vi "HW#1.vi"() -> ()   [LabVIEW 2018]
panel:
  out "Time":timestamp
  out "XY Graph":cluster{"X":dbl, "Y":dbl}[](graph)
  in  "File":path
  in  "Clear":bool
  in  "Plot Data":bool
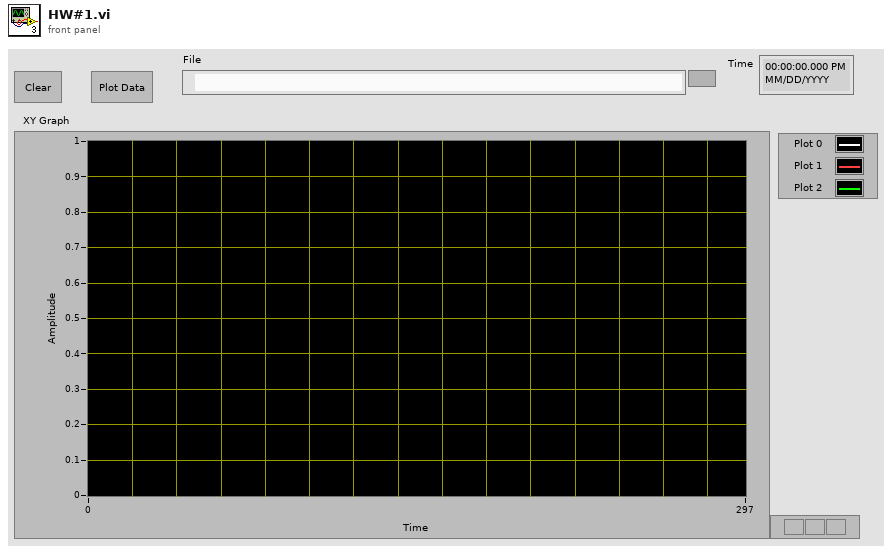
[diagram p1: front panel]
types:
  T1 = cluster{"Duration":u32, "State":bool, "Running":bool}
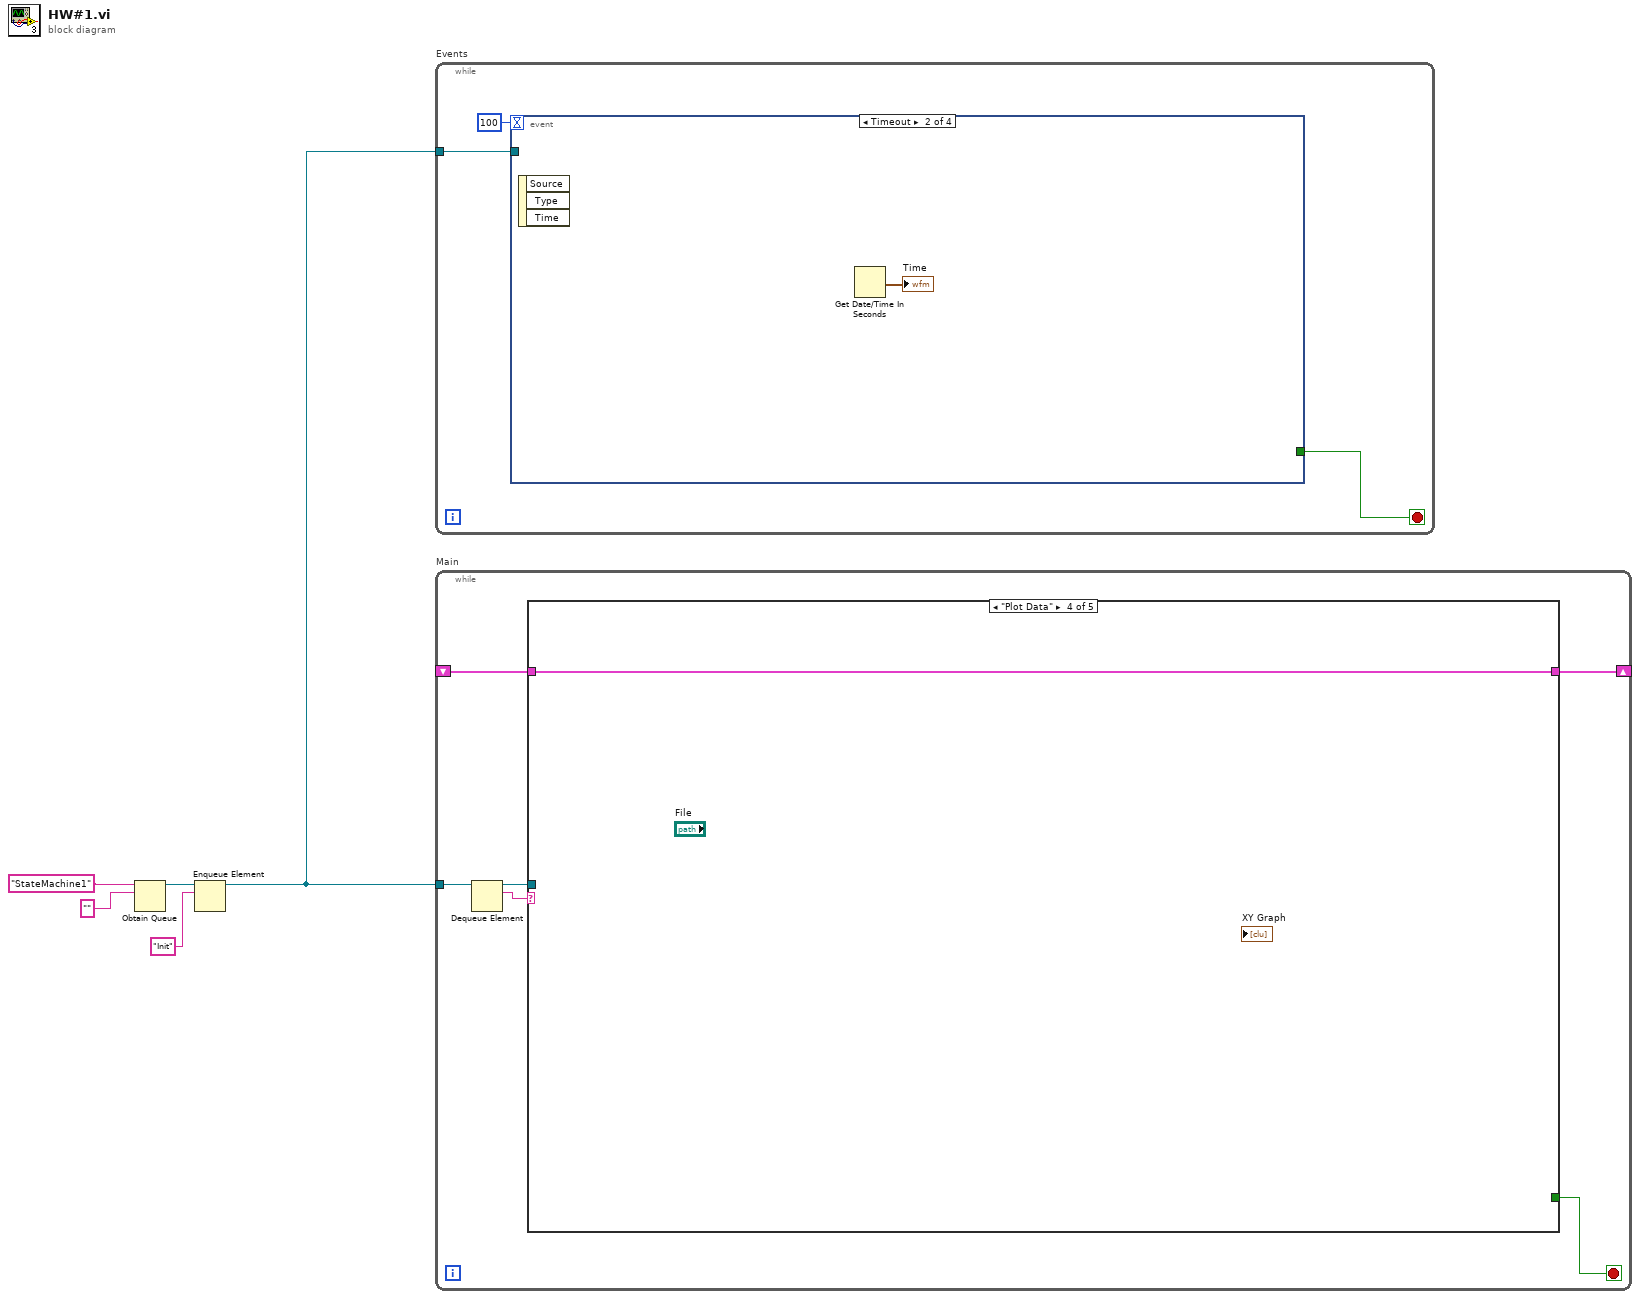
[diagram p0: block diagram]
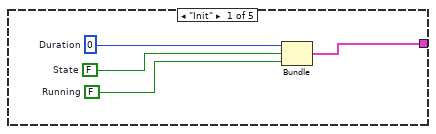
[diagram p2: hidden frame]
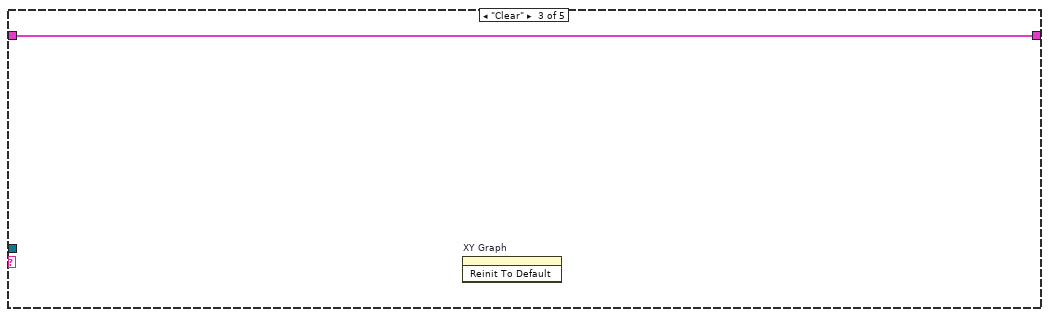
[diagram p4: hidden frame]
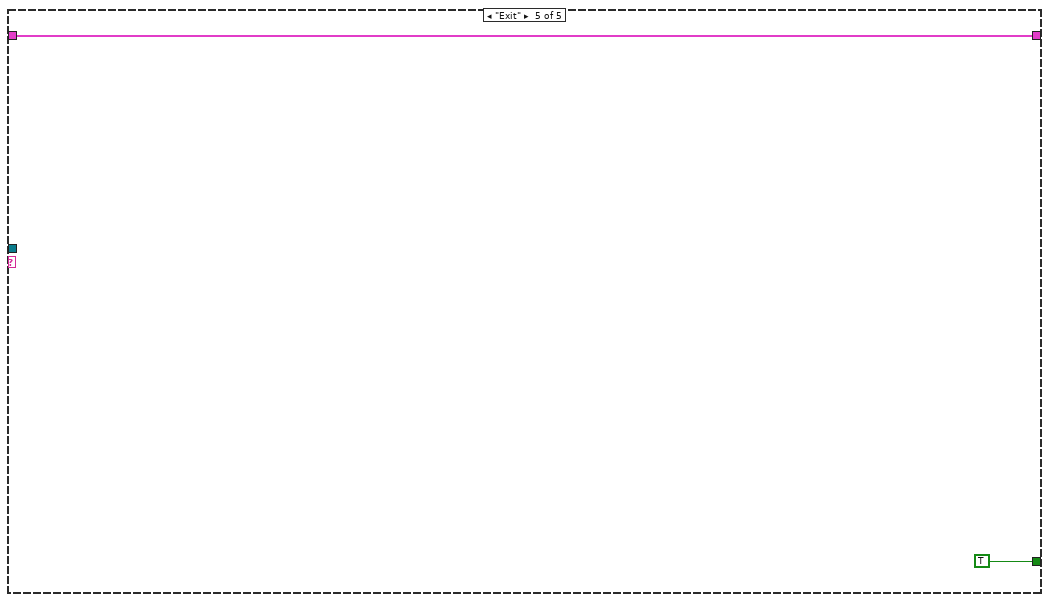
[diagram p5: hidden frame]
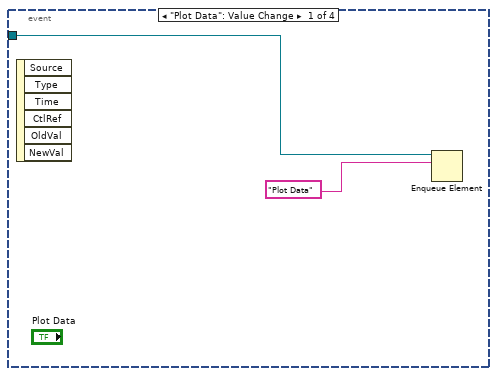
[diagram p6: hidden frame]
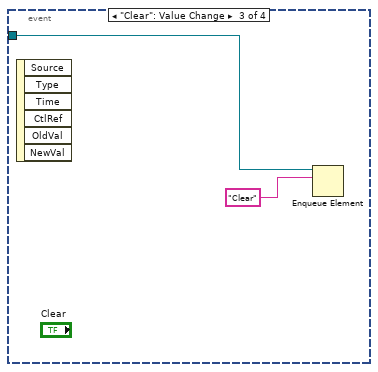
[diagram p7: hidden frame]
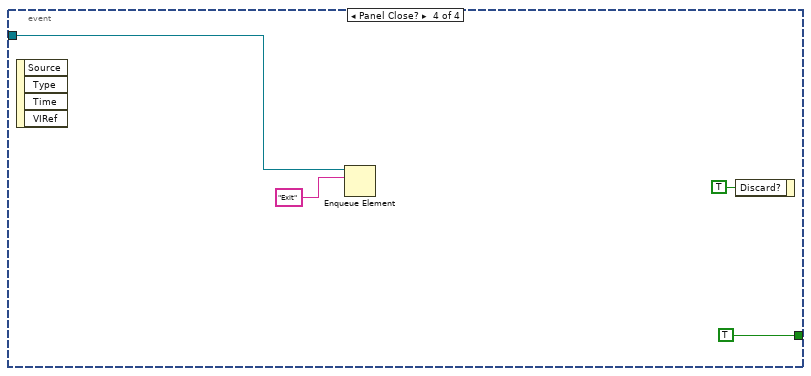
[diagram p8: hidden frame]
diagram:
  n1 = Obtain Queue(name (unnamed)="StateMachine1", element data type="") -> (queue out=w3:refnum<queue>)  [unwired: 3 in, 2 out]
  n2 = Enqueue Element(queue=w3, element="Init") -> (queue out=w2:refnum<queue>)  [unwired: 2 in, 2 out]
  n3 = while "Events" {
    tunnel: w2 -> [w8]
    stop <- w7 stop-if-true
    n4 = event shown="[1] Timeout" {
      selector: _ -> [_ _ _ _]
      dyn-events: _ -> [_ _ _ _]
      timeout: 100 -> [_ _ _ _]
      tunnel: w8 -> [w10 _ w13 w15]
      tunnel: [_ _ _ TRUE] -> w7
      event "Plot Data": Value Change {
        n5 = event-data() -> ()  [unwired: 1 in, 6 out]
        n6 = Enqueue Element(queue=w10, element="Plot Data") -> ()  [unwired: 2 in, 3 out]
      }
      event Timeout {
        n7 = event-data() -> ()  [unwired: 1 in, 3 out]
        n8 = Get Date/Time In Seconds() -> (seconds since 1Jan1904=→"Time":timestamp)
      }
      event "Clear": Value Change {
        n9 = event-data() -> ()  [unwired: 1 in, 6 out]
        n10 = Enqueue Element(queue=w13, element="Clear") -> ()  [unwired: 2 in, 3 out]
      }
      event Panel Close? {
        n11 = event-data() -> ()  [unwired: 1 in, 4 out]
        n12 = Enqueue Element(queue=w15, element="Exit") -> ()  [unwired: 2 in, 3 out]
        n13 = event-data("Discard?"=TRUE) -> ()  [unwired: 1 in, 1 out]
      }
    }
  }
  n14 = while "Main" {
    tunnel: w2 -> [w23]
    shift-right: [w18] -> _
    shift-left: _ -> [w19]
    stop <- w20 stop-if-true
    n15 = Dequeue Element(queue=w23) -> (queue out=w21:refnum<queue>, element=w22:string)  [unwired: 2 in, 2 out]
    n16 = case shown="\"Plot Data\"" w22 {
      tunnel: w21 -> [_ _ _ _ _]
      tunnel: [_ _ _ _ TRUE] -> w20
      tunnel: w19 -> [_ w28 w29 w30 w31]
      tunnel: [w27 w28 w29 w30 w31] -> w18
      frame "Init" {
        w24 = FALSE  # Running
        w25 = FALSE  # State
        w26 = u32 0  # Duration
        n17 = Bundle("Duration"=w26, "State"=w25, "Running"=w24) -> (w27:T1)  [unwired: 1 in]
      }
      frame Default {
      }
      frame "Clear" {
        n18 = invoke on="XY Graph" class="XYGraph (strict)" method="Reinit To Default"() -> ()  [unwired: 3 in, 3 out]
      }
      frame "Plot Data" {
      }
      frame "Exit" {
      }
    }
  }
